vi "Mod_OFDM_Set_Data_Source.vi"(0 "Configuration in":variant, 7 "Pool of Data Sources":T4 {"Register Initial State" format="%08x"}, 11 "error in":errorcluster) -> (4 "Configuration out":variant, 15 "error out":errorcluster)   [LabVIEW 2010]
uses:
  Controls(Type_DEf)/Pool of Data Source Control.ctl
  Controls(Type_DEf)/Attribute Data Types.ctl
  Controls(Type_DEf)/Configure Pulse Shaping.ctl
  Controls(Type_DEf)/Pool of Modulator Control.ctl
  Controls(Type_DEf)/Attribute Names.ctl
panel:
  in  "Attribute Data Types":T1={"Pulse Shaping"={"System Filter"={"TX Filter"=enum."none", "Alpha"=0.0, "filter length"=0}, "Modulation system parameters"={"samples per symbol (16)"=0}, "symbol rate (Hz)"=0.0}, "FRAME Table"=[], "OFDM Frame"=[], "Sub Carrier Selection"={"Sub Carrier Selection"=[], "OFDM Parameters"={"# of Sub Carrier"=0, "Length Of Cylic Prefix"=0}}, "Symbol Table"=[], "Symbol Pool"=[], "Pool of Modulators"=[], "Pool of Data Sources"=[], "Atribute Names"={"Data Source Pool"="Data Source Pool ", "Modulator Source Pool"="Modulator Source Pool ", "OFDM SYMBOL POOL"="OFDM SYMBOL POOL", "Symbol Table"="Symbol Table", "Sub Carrier Selection"="Sub Carrier Selection", "OFDM Frame"="OFDM Frame", "FRAME Table"="FRAME Table", "Pulse Shaping"="Pulse Shaping"}} {"Pool of Data Sources"."Register Initial State" format="%08x"; "Pulse Shaping"."symbol rate (Hz)" min=1.0 step=1.0 format="%.2p"; "Pulse Shaping"."Modulation system parameters"."samples per symbol (16)" step=2; "Pulse Shaping"."System Filter"."Alpha" min=0.0 max=1.0 step=0.05 format="%.2f"}
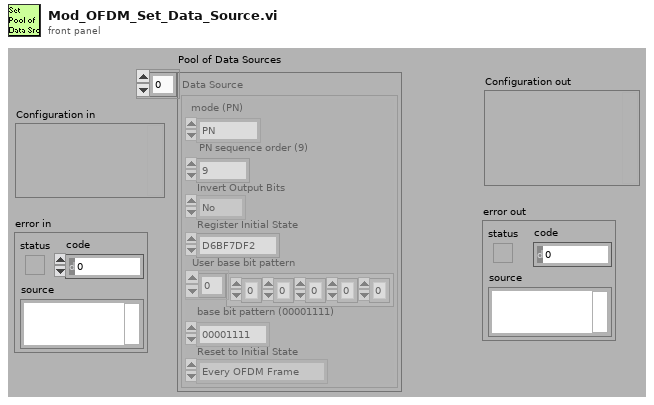
[diagram p1: front panel]
types:
  T1 = typedef "Attribute Data Types.ctl" = cluster{"Pulse Shaping":T2, "FRAME Table":string[][], "OFDM Frame":cluster{"Symbol Name":string, "# of Symbols":i32}[], "Sub Carrier Selection":cluster{"Sub Carrier Selection":cluster{"Sub Carrier":bool, "Data Source":u16, "Modulator":u16}[], "OFDM Parameters":cluster{"# of Sub Carrier":i32, "Length Of Cylic Prefix":i32}}, "Symbol Table":string[][], "Symbol Pool":string[], "Pool of Modulators":T3, "Pool of Data Sources":T4, "Atribute Names":T5}
  T2 = typedef "Configure Pulse Shaping.ctl" = cluster{"System Filter":cluster{"TX Filter":enum16{"none", "Raised Cosine", "Root Raised Cos"}, "Alpha":dbl, "filter length":i32}, "Modulation system parameters":cluster{"samples per symbol (16)":u32}, "symbol rate (Hz)":dbl}
  T3 = typedef "Pool of Modulator Control.ctl" = cluster{"M-QAM":enum16{"4", "16", "64", "256"}, "M-PSK":enum16{"2", "4", "8", "16", "32", "64", "128", "256"}, "Type of Modulation":enum16{"PSK", "QAM"}, " PSK":cluster{"differential PSK":enum16{"disable", "enable"}, "PSK type":enum16{"normal", "shifted", "offset"}}}[]
  T4 = typedef "Pool of Data Source Control.ctl" = cluster{"mode (PN)":enum16{"PN", "pattern", "user"}, "PN sequence order (9)":i32, "Invert Output Bits":enum16{"No", "Yes"}, "Register Initial State ":u32, "User base bit pattern":i8[], "base bit pattern (00001111)":enum16{"0", "1", "01", "0011", "00001111"}, "Reset to Initial State":enum16{"Every OFDM Frame", "Every OFDM Symbol", "Every Sub Carrier"}}[]
  T5 = typedef "Attribute Names.ctl" = cluster{"Data Source Pool":string, "Modulator Source Pool":string, "OFDM SYMBOL POOL":string, "Symbol Table":string, "Sub Carrier Selection":string, "OFDM Frame":string, "FRAME Table":string, "Pulse Shaping":string}
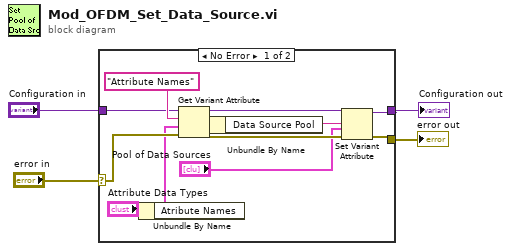
[diagram p0: block diagram]
diagram:
  n1 = case shown="No Error" "error in" {
    selector: "error in" -> [w13 w17]
    tunnel: "Configuration in" -> [w9 _]
    tunnel: [w16 _] -> w3
    tunnel: [w15 w17] -> w2
    frame No Error {
      n2 = Unbundle By Name("Attribute Data Types") -> ("Atribute Names"=w11:T5)
      n3 = Get Variant Attribute(Variant=w9, name="Attribute Names", default value (empty Variant)=w11, error in=w13) -> (duplicate Variant=w8:variant, value=w7:T5, error out=w12:errorcluster)  [unwired: 1 out]
      n4 = Unbundle By Name(w7) -> ("Data Source Pool"=w6:string)
      n5 = Set Variant Attribute(Variant=w8, name=w6, value="Pool of Data Sources", error in=w12) -> (Variant out=w16:variant, error out=w15:errorcluster)  [unwired: 1 out]
    }
    frame Error {
    }
  }
  "Configuration out" <- w3
  "error out" <- w2
